vi "cRIO A Main FPGA.vi"() -> ()   [LabVIEW 2012]
panel:
  out "Heartbeat":bool
  out "Encoder Position":fxp<+/-,32,32>
  out "Setpoint Pot":fxp<+/-,16,5>
  in  "Position Command (Deg)":fxp<+/-,20,5>
  in  "stop":bool
  in  "Count(mSec)":u32 caption="Loop Time (mSec)"
  # "Stepper Motor"
  # "Digital Servo Motor"
  # "Analog Servo Motor"
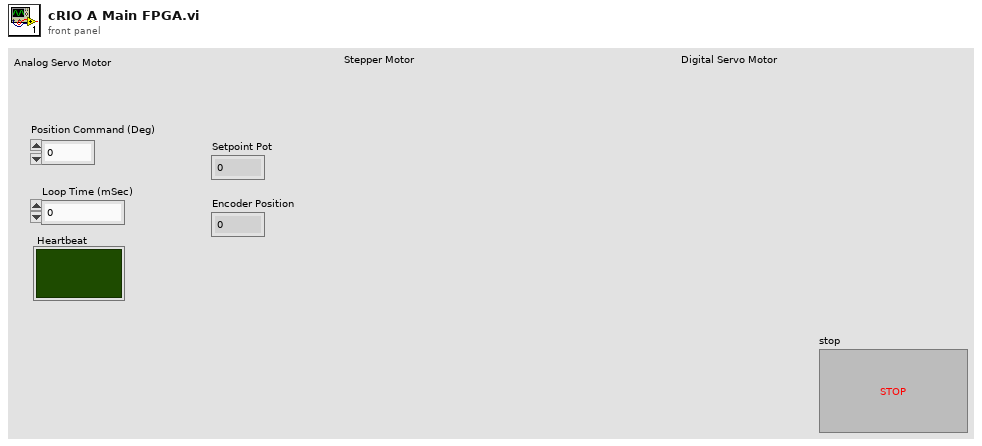
[diagram p1: front panel]
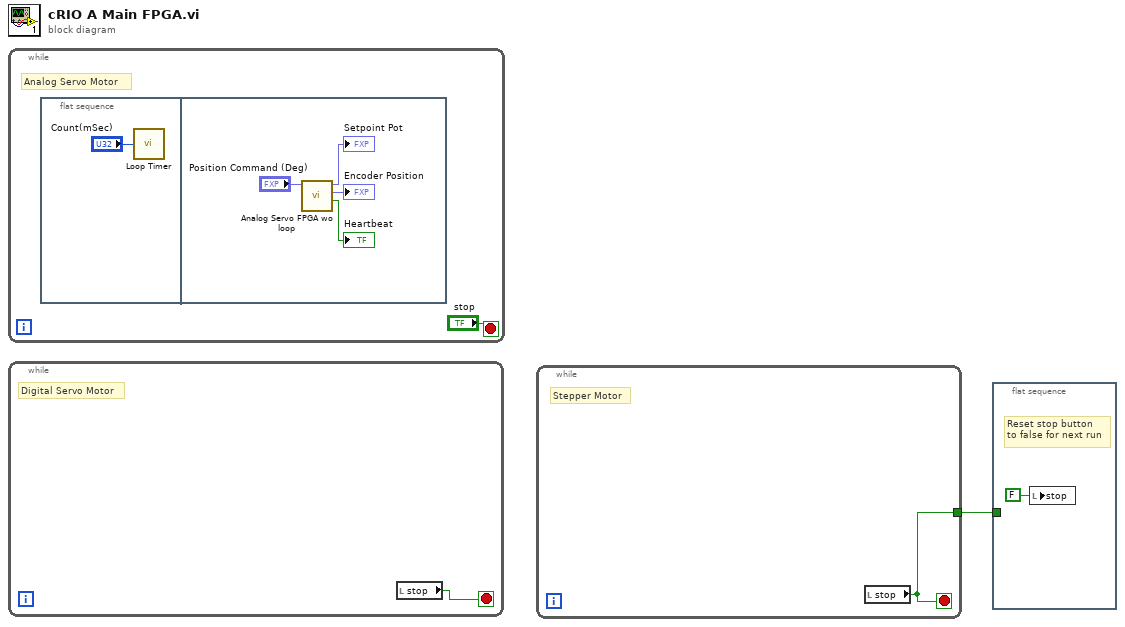
[diagram p0: block diagram]
diagram:
  n1 = while {
    stop <- "stop" stop-if-true
    # "Analog Servo Motor"
    n2 = flat-sequence {
      frame #0 {
        n3 = call "Loop Timer"("Count(mSec)"="Count(mSec)") -> ()  [unwired: 1 out]
      }
      frame #1 {
        n4 = call "Analog Servo FPGA wo loop.vi"("Command Voltage"="Position Command (Deg)") -> ("Heartbeat"=→"Heartbeat":bool, "Position Out"=→"Encoder Position":fxp<+/-,32,32>, "Setpoint Pot"=→"Setpoint Pot":fxp<+/-,16,5>)  [unwired: 8 in]
      }
    }
  }
  n5 = while {
    stop <- w8 stop-if-true
    # "Digital Servo Motor"
    n6 = local read "stop"() -> (w8:bool)
  }
  n7 = while {
    tunnel: [w9] -> w1
    stop <- w9 stop-if-true
    # "Stepper Motor"
    n8 = local read "stop"() -> (w9:bool)
  }
  n9 = flat-sequence {
    tunnel: w1 -> [_]
    frame #0 {
      # "Reset stop button\nto false for next run"
      n10 = local write "stop"(FALSE ("stop")) -> ()
    }
  }
